vi "get Data Read.vi"(7 "data_pos":u16, 9 "data_length":u16, 10 "protocol_version":i32, 11 "port_num":i32) -> (3 "function return":u32)   [LabVIEW 2015, in "dxl_x86_c.lvlib"]
doc: "WINDECLSPEC uint32_t getDataRead (int port_num, int protocol_version, uint16_t data_length, uint16_t data_pos);"
uses:
  dxl_x86_c.lvlib
  dxl_x86_c.dll
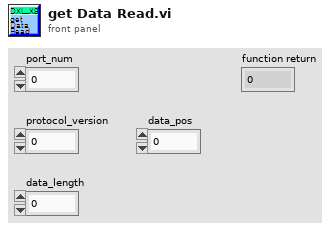
[diagram p1: front panel]
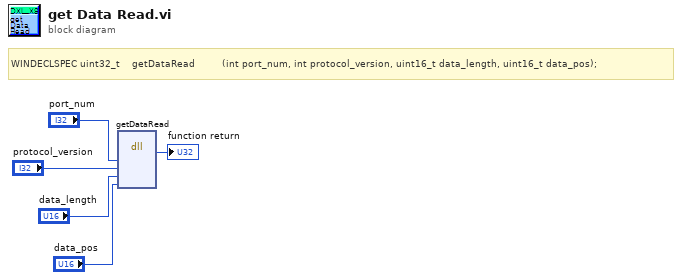
[diagram p0: block diagram]
diagram:
  # "WINDECLSPEC uint32_t    getDataRead         (int port_num, int protocol_version, uint16_t data_length, uint16_t data_pos);"
  n1 = dll-call lib="C:/Users/Platform/Desktop/LabVIEW/dxl_x86_c.lvlib/dxl_x86_c.*" fn="getDataRead"("port_num"="port_num", "protocol_version"="protocol_version", "data_length"="data_length", "data_pos"="data_pos") -> (→"function return":u32)  [unwired: 7 in, 2 out]
